vi "configuration_pv.vi"(9 "framerate":u8=30, 10 "height":u16=1080, 11 "width":u16=1920) -> (3 "configuration_pv":T1={"chunk"=4096, "mode"=1, "_reserved_0"=0, "width"=1920, "height"=1080, "framerate"=30, "_reserved_1"=0, "divisor"=1, "profile"=3, "level"=255, "decoded format"=2, "bitrate"=0, "options_size"=-1, "options_data"=0, "_reserved_2"=0})   [LabVIEW 2023]
panel:
  in  "configuration_pv":T1={"chunk"=4096, "mode"=1, "_reserved_0"=0, "width"=1920, "height"=1080, "framerate"=30, "_reserved_1"=0, "divisor"=1, "profile"=3, "level"=255, "decoded format"=2, "bitrate"=0, "options_size"=-1, "options_data"=0, "_reserved_2"=0}
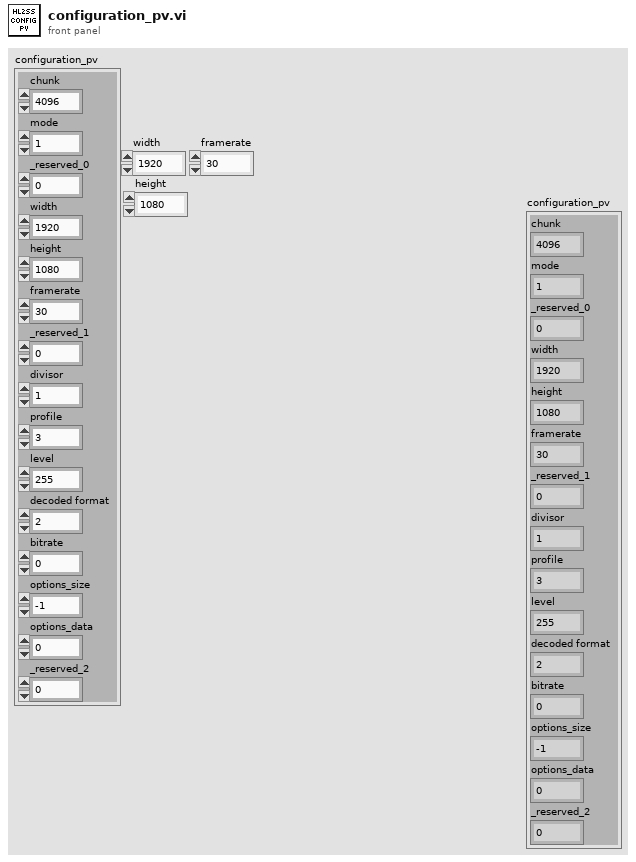
[diagram p1: front panel]
types:
  T1 = cluster{"chunk":u64, "mode":u8, "_reserved_0":u8, "width":u16, "height":u16, "framerate":u8, "_reserved_1":u8, "divisor":u8, "profile":u8, "level":u8, "decoded format":u8, "bitrate":u32, "options_size":i64, "options_data":u64, "_reserved_2":u64}
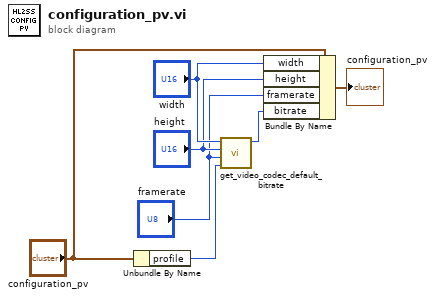
[diagram p0: block diagram]
diagram:
  n1 = Unbundle By Name("configuration_pv") -> ("profile"=w3:u8)
  n2 = call "get_video_codec_default_bitrate.vi"("profile"=w3, "framerate"="framerate", "height"="height", "width"="width") -> ("bitrate"=w2:u32)  [unwired: 7 in]
  n3 = Bundle By Name(cluster="configuration_pv", "width"="width", "height"="height", "framerate"="framerate", "bitrate"=w2) -> (→"configuration_pv":T1)
